vi "Set Platform Application Attributes.vi"(8 "error in (no error)":errorcluster, 10 "Platform Application Attributes":T1[](array[typedef]), 11 "Platform Application in":refnum<class "Platform Application.lvclass">) -> (0 "error out":errorcluster, 3 "Platform Application out":refnum<class "Platform Application.lvclass">)   [LabVIEW 2015, in "NI_AWS_SNS.lvlib" / "Platform Application.lvclass"]
uses:
  Platform Application.lvclass
  Application Attribute Value Pair.ctl
  Application Attribute.ctl
  Core/HTTP Request/Request Options.ctl
  Core/HTTP Request/Name Value Pair.ctl
  Core/ARN/ARN.lvclass/ARN.ctl
  Core/ARN/Read ARN.vi
  Core/HTTP Request/HTTP Request.lvclass
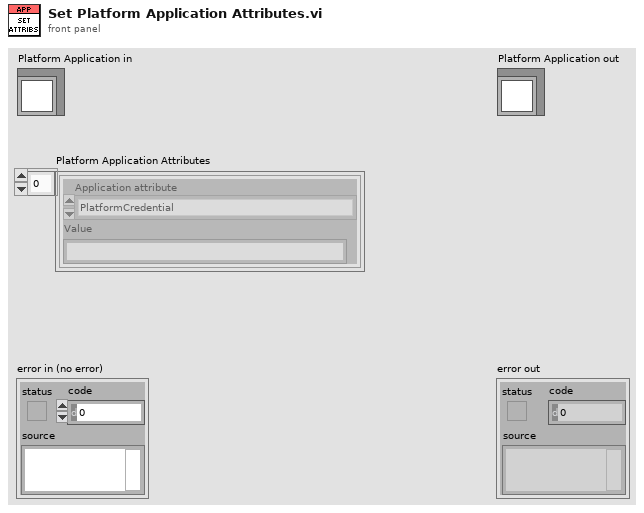
[diagram p1: front panel]
types:
  T1 = typedef "NI_AWS_SNS.lvlib/Platform Application.lvclass/Application Attribute Value Pair.ctl" = cluster{"Application attribute":T2, "Value":string}
  T2 = typedef "NI_AWS_SNS.lvlib/Platform Application.lvclass/Application Attribute.ctl" = enum16{"PlatformCredential", "PlatformPrincipal", "EventEndpointCreated", "EventEndpointDeleted", "EventEndpointUpdated", "EventDeliveryFailure", "SuccessFeedbackRoleArn", "FailureFeedbackRoleArn", "SuccessFeedbackSampleRate"}
  T3 = typedef "NI_AWS_Core.lvlib/HTTP Request.lvclass/Name Value Pair.ctl" = cluster{"name":string, "value":string}
  T4 = typedef "NI_AWS_Core.lvlib/HTTP Request.lvclass/Request Options.ctl" = cluster{"request headers":T3[], "request parameters":T3[], "request body":string}
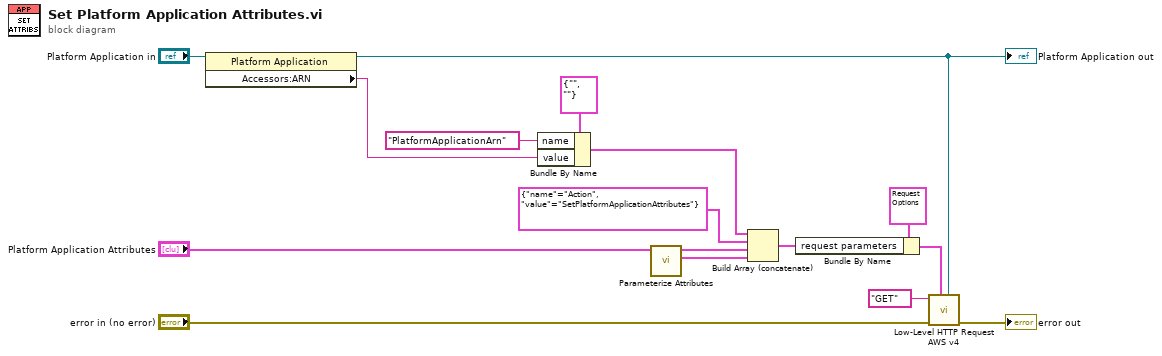
[diagram p0: block diagram]
diagram:
  n1 = property class="Platform Application"(reference="Platform Application in") -> (reference out=w6:refnum<class "Platform Application.lvclass">, "Accessors:ARN"=w9:string)  [unwired: 1 in, 1 out]
  "Platform Application out" <- w6
  n2 = Bundle By Name(cluster=T3 {"name"="", "value"=""} ("element"), "name"="PlatformApplicationArn", "value"=w9) -> (w8:T3)
  n3 = call "Parameterize Attributes.vi"("Platform Application Attributes"="Platform Application Attributes") -> ("values"=w4:T3[], "attributes"=w5:T3[])  [unwired: 9 in]
  n4 = Build Array (concatenate)(w8, T3 {"name"="Action", "value"="SetPlatformApplicationAttributes"} ("Cluster"), w5, w4) -> (w12:T3[])
  n5 = Bundle By Name(cluster=T4 {"request headers"=[], "request parameters"=[{"name"="Action", "value"="ListQueues"}], "request body"=""} ("Request Options"), "request parameters"=w12) -> (w14:T4)
  n6 = call "Low-Level HTTP Request AWS v4.vi"("AWS Core"=w6, "Request Options"=w14, "error in (no error)"="error in (no error)", "HTTP-Verb"="GET") -> ("error out"=→"error out":errorcluster)  [unwired: 5 in, 2 out]
